vi "p2.vi"() -> ()   [LabVIEW 2021, in "d12.lvlib"]
uses:
  d12.lvlib
  AOC/AOC.lvlib
panel:
  out "vertex":i32
  out "XY Graph":cluster{"row":i32, "col":i32}[](graph)
  out "Answer":i32
  in  "Example":string="Sabqponm\nabcryxxl\naccszExk\nacctuvwj\nabdefghi"
  in  "Example":bool
  out "Height Map":i16[][](graph)
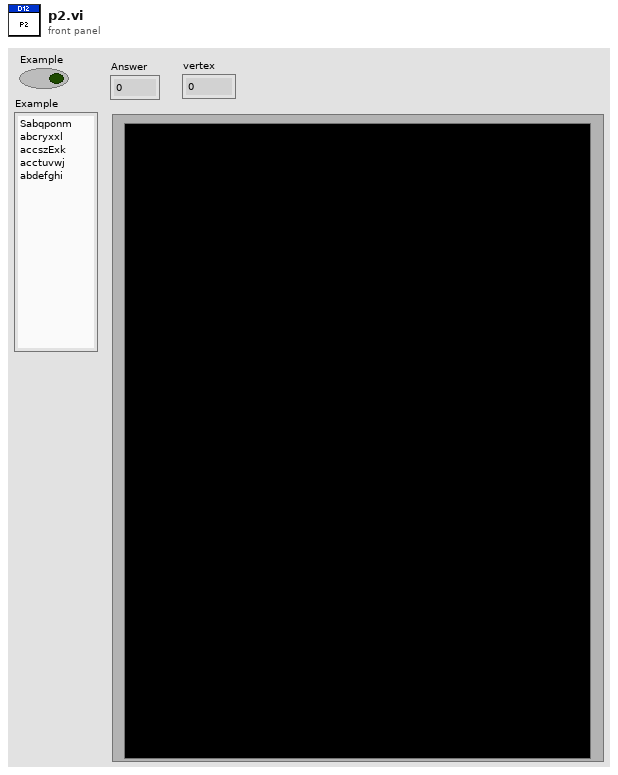
[diagram p1: front panel]
types:
  T1 = map{cluster{"row":i32, "col":i32}, cluster{"Height":i16, "Parent":cluster{"row":i32, "col":i32}, "Explored?":bool}}
  T2 = cluster{"Height":i16, "Parent":cluster{"row":i32, "col":i32}, "Explored?":bool}
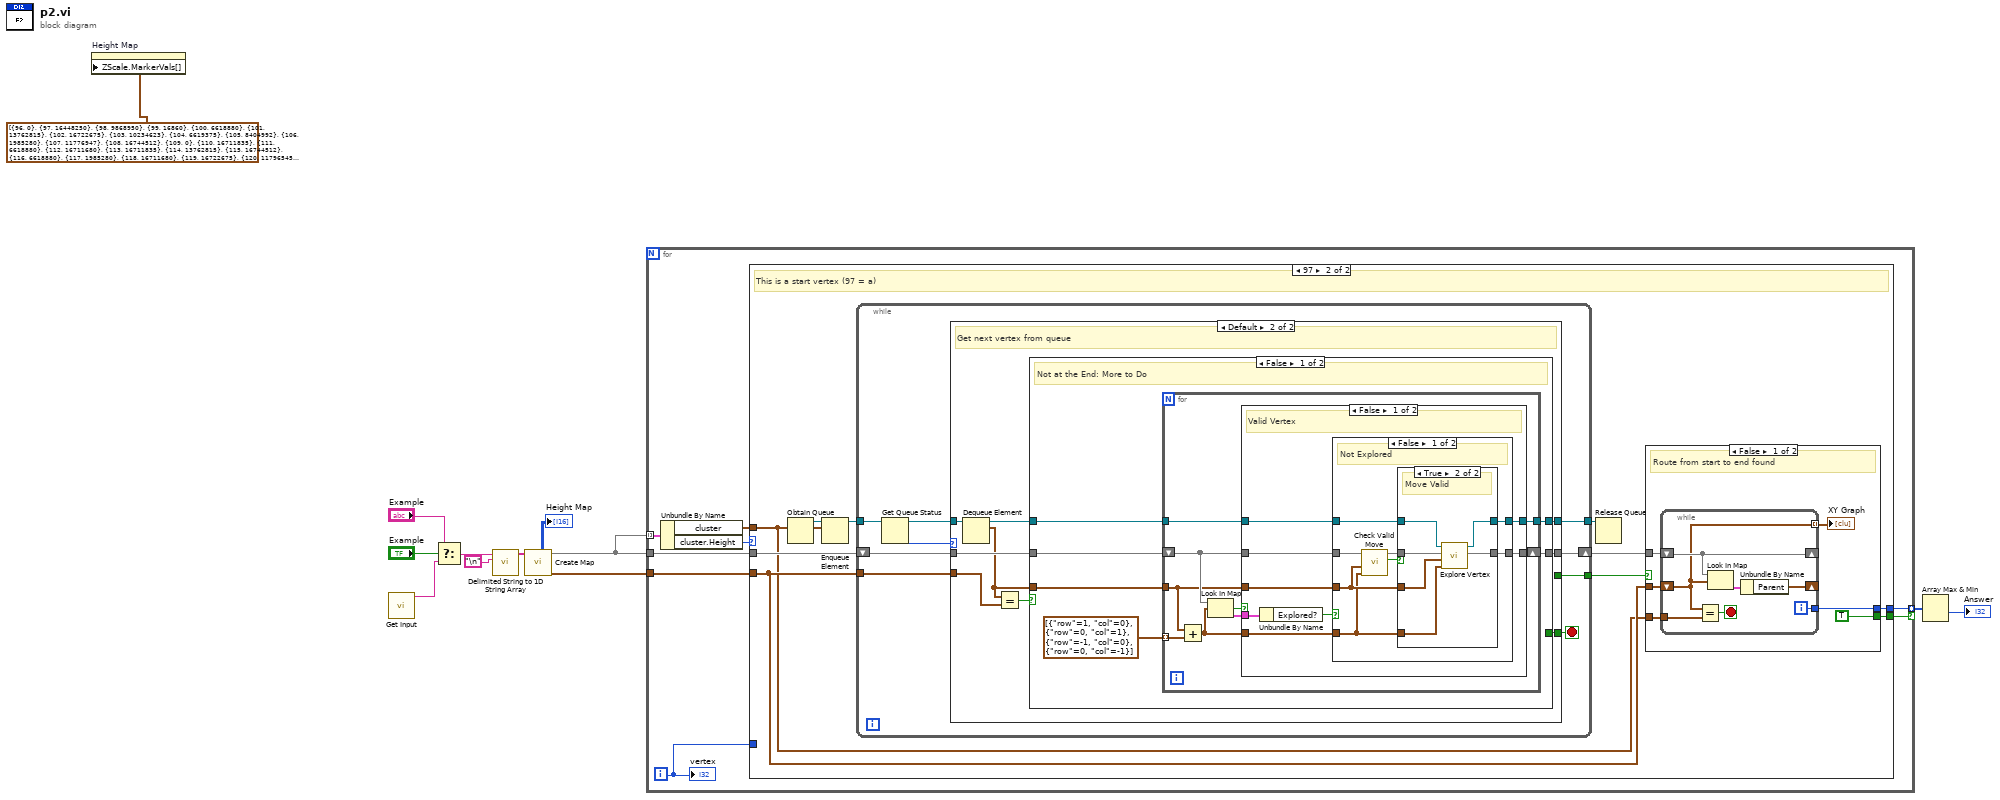
[diagram p0: block diagram]
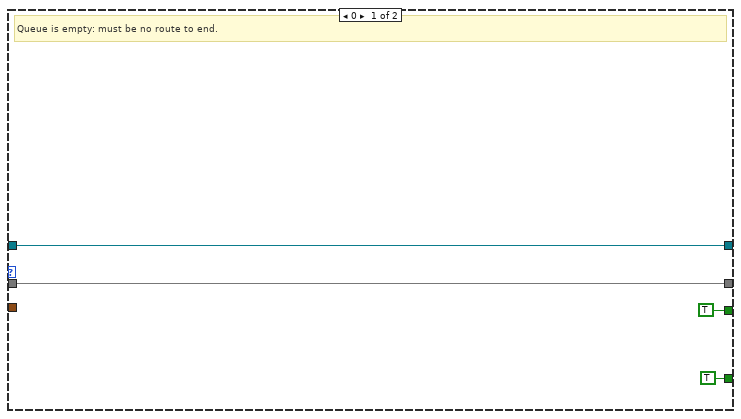
[diagram p3: hidden frame]
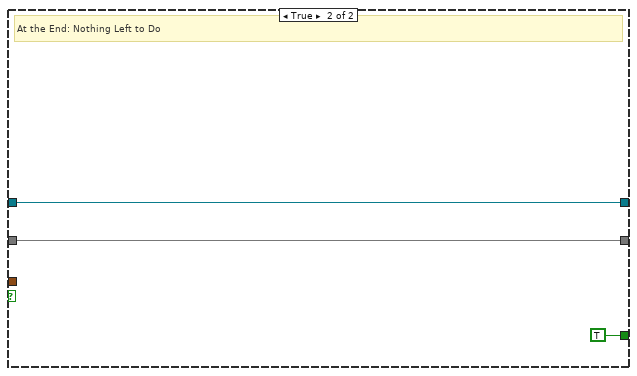
[diagram p7: hidden frame]
diagram:
  n1 = property on="Height Map" class="IntGraph (strict)"("ZScale.MarkerVals[]"=cluster{i16, u32}[] [{96, 0}, {97, 16448250}, {98, 9868950}, {99, 16860}, {100, 6618880}, {101, 13762815}, {102, 16722675}, {103, 10234623}, {104, 6619375}, {105, 8404992}, {106, 1985280}, {107, 11776947}, {108, 16744512}, {109, 0}, {110, 16711835}, {111, 6618880}, {112, 16711680}, {113, 16711835}, {114, 13762815}, {115, 16744512}, {116, 6618880}, {117, 1985280}, {118, 16711680}, {119, 16722675}, {120, 11796545}, {121, 7171459}, {122, 7171459}, {123, 0}] ("Z Scale.Marker Values[]")) -> ()  [unwired: 2 in, 2 out]
  n2 = call "Get Input.vi"() -> ("Input"=w12:string)  [unwired: 11 in]
  n3 = Select(t="Example", s="Example", f=w12) -> (s? t:f=w11:string)
  n4 = call <vilib>:"Delimited String to 1D String Array.vi"("delimiter"="\n", "delimited string"=w11) -> ("string array"=w4:string[])  [unwired: 9 in]
  n5 = call "Create Map.vi"("input"=w4) -> ("End"=w1:cluster{"row":i32, "col":i32}, "Map"=w2:T1, "Heights"=→"Height Map":i16[][])  [unwired: 7 in, 1 out]
  n6 = for {
    tunnel: w2 -> [w20]
    tunnel: [w19] -> w6 mode=indexing if=w13
    tunnel: w2 -> [w18] mode=indexing
    tunnel: w1 -> [w14]
    i -> [w15]
    n7 = Unbundle By Name(w18) -> ("cluster"=w17:cluster{"row":i32, "col":i32}, "cluster.Height"=w16:i16)
    n8 = case shown="97" w16 {
      tunnel: w20 -> [_ w26]
      tunnel: [_ w30] -> w19
      tunnel: w17 -> [_ w21]
      tunnel: w15 -> [_ _]
      tunnel: w14 -> [_ w22]
      tunnel: [_ w23] -> w13
      frame 0, Default {
      }
      frame 97 {
        # "This is a start vertex (97 = a)"
        n9 = Obtain Queue(element data type=w21) -> (queue out=w29:refnum<queue>)  [unwired: 4 in, 2 out]
        n10 = Enqueue Element(queue=w29, element=w21) -> (queue out=w28:refnum<queue>)  [unwired: 2 in, 2 out]
        n11 = while {
          shift-right: [w37] -> w25
          shift-left: w26 -> [w39]
          tunnel: w22 -> [w38]
          tunnel: w28 -> [w35]
          tunnel: [w34] -> w27
          tunnel: [w33] -> w24
          stop <- w32 stop-if-true
          n12 = Get Queue Status(queue=w35) -> (queue out=w36:refnum<queue>, # elements in queue=w31:i32)  [unwired: 2 in, 6 out]
          n13 = case shown="Default" w31 {
            tunnel: w39 -> [w42 w52]
            tunnel: w38 -> [_ w51]
            tunnel: [w42 w49] -> w37
            tunnel: w36 -> [w43 w46]
            tunnel: [w43 w45] -> w34
            tunnel: [TRUE _] -> w33
            tunnel: [TRUE w44] -> w32
            frame 0 {
              # "Queue is empty: must be no route to end."
            }
            frame Default {
              # "Get next vertex from queue"
              n14 = Dequeue Element(queue=w46) -> (queue out=w47:refnum<queue>, element=w48:cluster{"row":i32, "col":i32})  [unwired: 2 in, 2 out]
              n15 = Equal?(x=w48, y=w51) -> (x = y?=w50:bool)
              n16 = case shown="False" w50 {
                tunnel: w52 -> [w55 w98]
                tunnel: w48 -> [w54 _]
                tunnel: [w58 w98] -> w49
                tunnel: w47 -> [w56 w97]
                tunnel: [w53 w97] -> w45
                tunnel: [_ TRUE] -> w44
                frame False {
                  # "Not at the End: More to Do"
                  n17 = for {
                    tunnel: w54 -> [w59]
                    shift-right: [w64] -> w58
                    shift-left: w55 -> [w65]
                    tunnel: cluster{"row":i32, "col":i32}[] [{"row"=1, "col"=0}, {"row"=0, "col"=1}, {"row"=-1, "col"=0}, {"row"=0, "col"=-1}] ("element") -> [w67] mode=indexing
                    tunnel: w56 -> [w62]
                    tunnel: [w60] -> w53
                    n18 = Add(x=w59, y=w67) -> (x+y=w61:cluster{"row":i32, "col":i32})
                    n19 = Look In Map(map=w65, key=w61) -> (key not found?=w66:bool, value=w63:T2)  [unwired: 1 in]
                    n20 = case shown="False" w66 {
                      tunnel: w65 -> [w70 w95]
                      tunnel: [w69 w95] -> w64
                      tunnel: w63 -> [w74 _]
                      tunnel: w62 -> [w71 w94]
                      tunnel: w59 -> [w73 _]
                      tunnel: w61 -> [w72 _]
                      tunnel: [w68 w94] -> w60
                      frame False {
                        # "Valid Vertex"
                        n21 = Unbundle By Name(w74) -> ("Explored?"=w75:bool)
                        n22 = case shown="False" w75 {
                          tunnel: w73 -> [w80 _]
                          tunnel: w72 -> [w79 _]
                          tunnel: w71 -> [w83 w92]
                          tunnel: w70 -> [w76 w93]
                          tunnel: [w82 w93] -> w69
                          tunnel: [w81 w92] -> w68
                          frame False {
                            # "Not Explored"
                            n23 = call "Check Valid Move.vi"("Vertex"=w79, "Parent"=w80, "Map in"=w76) -> ("Valid Move?"=w78:bool, "Map out"=w77:T1)  [unwired: 7 in]
                            n24 = case shown="True" w78 {
                              tunnel: w80 -> [_ w91]
                              tunnel: w83 -> [w84 w90]
                              tunnel: w79 -> [_ w86]
                              tunnel: w77 -> [w85 w89]
                              tunnel: [w85 w88] -> w82
                              tunnel: [w84 w87] -> w81
                              frame False {
                                # "Move Invalid"
                              }
                              frame True {
                                # "Move Valid"
                                n25 = call "Explore Vertex.vi"("Vertex"=w86, "Parent"=w91, "Map in"=w89, "Queue in"=w90) -> ("Map out"=w88:T1, "Queue out"=w87:refnum<queue>)  [unwired: 6 in]
                              }
                            }
                          }
                          frame True {
                            # "Explored"
                          }
                        }
                      }
                      frame True {
                        # "Invalid Vertex"
                      }
                    }
                  }
                }
                frame True {
                  # "At the End: Nothing Left to Do"
                }
              }
            }
          }
        }
        n26 = Release Queue(queue=w27) -> ()  [unwired: 2 in, 3 out]
        n27 = case shown="False" w24 {
          tunnel: w25 -> [w104 _]
          tunnel: [w100 _] -> w30
          tunnel: w22 -> [w102 _]
          tunnel: w21 -> [w101 _]
          tunnel: [TRUE _] -> w23
          frame False {
            # "Route from start to end found"
            n28 = while {
              shift-right: [w111] -> _
              shift-left: w104 -> [w111]
              shift-right: [w109] -> _
              shift-left: w102 -> [w105]
              tunnel: w101 -> [w108]
              tunnel: [w106] -> w100
              tunnel: [w105] -> w103 mode=indexing
              i -> [w106]
              stop <- w107 stop-if-true
              n29 = Equal?(x=w105, y=w108) -> (x = y?=w107:bool)
              n30 = Look In Map(map=w111, key=w105) -> (value=w110:T2)  [unwired: 1 in, 1 out]
              n31 = Unbundle By Name(w110) -> ("Parent"=w109:cluster{"row":i32, "col":i32})
            }
            "XY Graph" <- w103
          }
          frame True {
            # "Route from start to end not found"
          }
        }
      }
    }
    "vertex" <- w15
  }
  n32 = Array Max & Min(array=w6) -> (min value=→"Answer":i32)  [unwired: 3 out]
